vi "MODAQ RD v1.0 Main (DAQmx).vi"() -> ()   [LabVIEW 2019]
uses:
  Sub-VIs/Globals and Definitions/System Message.ctl
  <vilib>/Platform/TimedLoop/XDataNode/timing_clust.ctl
  <vilib>/Platform/TimedLoop/XDataNode/nitl_modes.ctl
  <vilib>/Platform/TimedLoop/XDataNode/wakeup.ctl
  Sub-VIs/Globals and Definitions/RT Globals RD v1.0.vi
  Sub-VIs/Globals and Definitions/Initialization Globals.vi
  Sub-VIs/Globals and Definitions/Control Globals RD v1.0.vi
  <instrlib>/niSync/niSync.llb/niSync Initialize (Default).vi
  <userlib>/_OpenG.lib/comparison/comparison.llb/U32 Changed__ogtk.vi
  <vilib>/Platform/TimedLoop/XDataNode/XDataNode.xnode
  <resource>/objmgr/nisysapi.rc
  <vilib>/Platform/TimedLoop/XDataNode/XDNodeRunTimeDep.lvlib
  <vilib>/nisyscfg/nisyscfg.lvlib
panel:
  in  "Port State":i32(ring)=3 items=["Disabled"=3, "Master"=6, "Passive"=7, "Slave"=9]
  out "Not SavingTDMS Data":bool
  out "Saving TDMS Data":bool=TRUE
  out "TDMS Recording Mode":string="Interval"
  out "Ring":u16(ring) items=["Fix Unavailable", "2D GNSS Fix", "3D GNSS Fix", "SBAS GNSS Fix", "Differential GNSS Fix", "Omnistar/Starfire GNSS fix", "RTK Float GNSS fix", "RTK Fixed GNSS fix"]
  out "GNSS Fix Status":i16
  out "PTP Time Server Found":bool
  out "satellites available":u8
  out "CPU Utili Label":string="CPU Utilization (%)"
  out "CPU Utilization %":string="3.4"
  out "RAM Free Label":string="RAM Free (%)"
  out "RAM Free (%)":string="88.0"
  out "Disk % Label":string="Disk Free (%)"
  out "Disk Free (%)":string="99.6"
  out "Disk Free Label":string="Disk Free (GB)"
  out "Disk Free (GB)":string="1992.8"
  out "Errors":errorcluster
  in  "STOP":bool
  out "Uptime String":string="Uptime:   0d  0h  0m"
  out "date/time string":string="Oct 26, 2023    12:39:58 UTC"
  out "Heading":string="Heading: 0.0°"
  out "Offset Distance":string="Offset: 11303146.1m"
  out "Current Position":string="Current Position: 0.000, 0.000"
  # "3 Phase Data Save"
  # "GPS Timekeeper Status"
  # "GPS Position Status"
  # "MODAQ\nNREL       RD v1.0"
  # "Public Reference\nDesign"
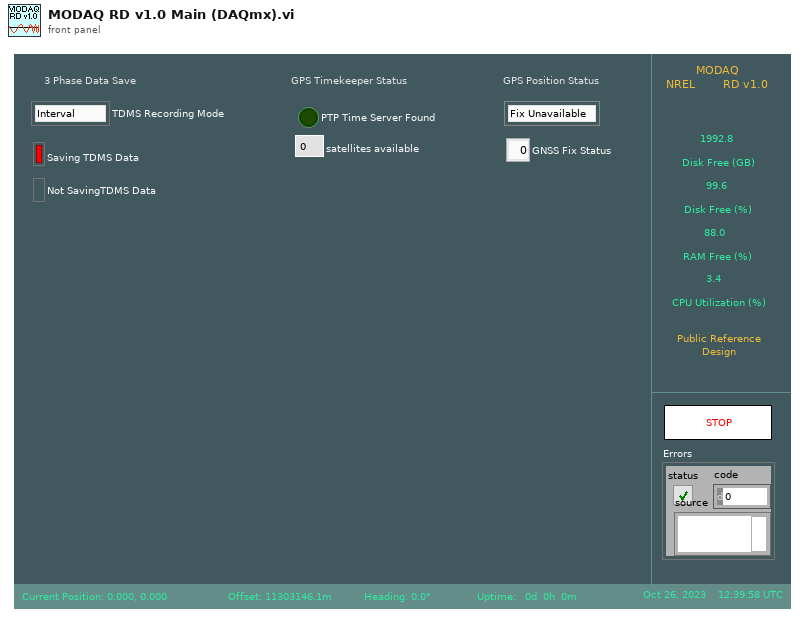
[diagram p1: front panel]
types:
  T1 = typedef "System Message.ctl" = cluster{"Message Tag":string, "Message Body":string, "Snooze Time (s)":dbl, "Snooze Alert?":bool, "Log Event?":bool, "Send Email":i32}
  T2 = typedef "All Tab Controls RDv1.0.ctl" = cluster{"Watch Circle":T3, "FTP and AWS":T4, "Email Settings":T5, "Summary File":T6, "File Settings":T7, "Watchdog":T9, "PowGrp0":T10, "Scaling Factors Grp0":dbl[], "PowGrp0 Sampling":cluster{"PowGrp0 sample rate [Hz]":dbl, "PowGrp0 samples per channel":i32}, "Stbd 3 Phase Voltage Scaling":dbl[], "Stbd 3 Phase Current Scaling":dbl[]}
  T3 = typedef "Watch Circle.ctl" = cluster{"Set Point Lat (dd)":dbl, "Set Point Lon (dd)":dbl, "Yellow Alert Radius (m)":dbl, "Red Alert Radius (m)":dbl, "AWOL Radius (m)":dbl, "Yellow Alert Snooze (min)":dbl, "Red Alert Snooze (min)":dbl, "AWOL Radius Snooze (min)":dbl}
  T4 = typedef "AWS and FTP.ctl" = cluster{"AWS Access Key":string, "AWS Secret Key":string, "AWS Bucket":string, "Enable AWS Upload (Summary)":bool, "Enable FTP Upload":bool, "FTP Host":string, "FTP User":string, "FTP Password":string, "Destination write path (pos)":string, "Local file path (pos)":string, "Summary  Upload Interval pos (min)":i32, "Delete Local File After Upload":bool, "Destination write path (pow)":string, "Local file path (pow)":string, "Summary Upload Interval pow (min)":i32, "Enable AWS Upload (TDMS)":bool}
  T5 = typedef "Email Settings.ctl" = cluster{"Enable Alerts":bool, "Distribution List (comma separated) 1":string, "Distribution List (comma separated) 2":string, "Sender Email":string, "SMTP":string, "Username":string, "Password":string}
  T6 = typedef "Summary File.ctl" = cluster{"Enable CSV":bool, "CSV Averaging Time (Sec)":i32, "CSV Loop Delay (ms)":i32}
  T7 = typedef "File Settings.ctl" = cluster{"Config File Path":string, "Data Folder Path":string, "Raw Mode":string, "Raw Interval (min)":i32, "Raw Sampling Time (min)":i32, "TDMS File Write Interval":T8, "Default Filename":path, "Enable TDMS Save (3ph only)":bool}
  T8 = typedef "Enum_FileNewInterval.ctl" = enum16{"10 Min", "Hourly", "Daily", "Weekly", "Monthly"}
  T9 = typedef "Watchdog.ctl" = cluster{"Watchdog Period (ms)":u32, "Reset System on WD timeout":bool, "Enable RT Watchdog":bool}
  T10 = typedef "TDMS Constants.ctl" = cluster{"Channel Names":string[], "Channel Units":string[], "TDMS File Suffix":string, "Channel Datatype":string[]}
  T11 = typedef "XDNodeRunTimeDep.lvlib/timing_clust.ctl" = cluster{"Expected End [f-1]":u64, "Actual End [f-1]":u64, "Finished Late? [f-1]":bool, "Expected End [i-1]":u64, "Actual End [i-1]":u64, "Finished Late? [i-1]":bool, "Expected Start [i]":u64, "Actual Start [i]":u64, "Expected Start [f]":u64, "Actual Start [f]":u64, "Source Name":string, "Structure Name":string, "Period":i64, "Deadline":i64, "Offset":i64, "Start":i64, "Priority":i32, "Timeout":i32, "Mode":T12, "Wakeup Reason":T13, "Error":errorcluster, "Source Type":string, "Secondary Source Type":string, "Global End Time":u64, "Global Start Time":u64, "Frame Duration":u64, "Iteration Duration":u64, "Assigned CPU":i32, "I/O Scan Engine Mode":u32}
  T12 = typedef "XDNodeRunTimeDep.lvlib/nitl_modes.ctl" = enum32{"No Change", "Process missed periods, maintain original phase", "Discard missed periods, maintain original phase", "Process missed periods, ignore original phase", "Discard missed periods, ignore original phase"}
  T13 = typedef "XDNodeRunTimeDep.lvlib/wakeup.ctl" = enum32{"Normal", "Aborted", "Asynchronous wakeup", "Timing source error", "Timed loop error", "Timeout"}
  T14 = enum16{"open", "replace", "create", "open or create", "replace or create", "replace or create with confirmation"}
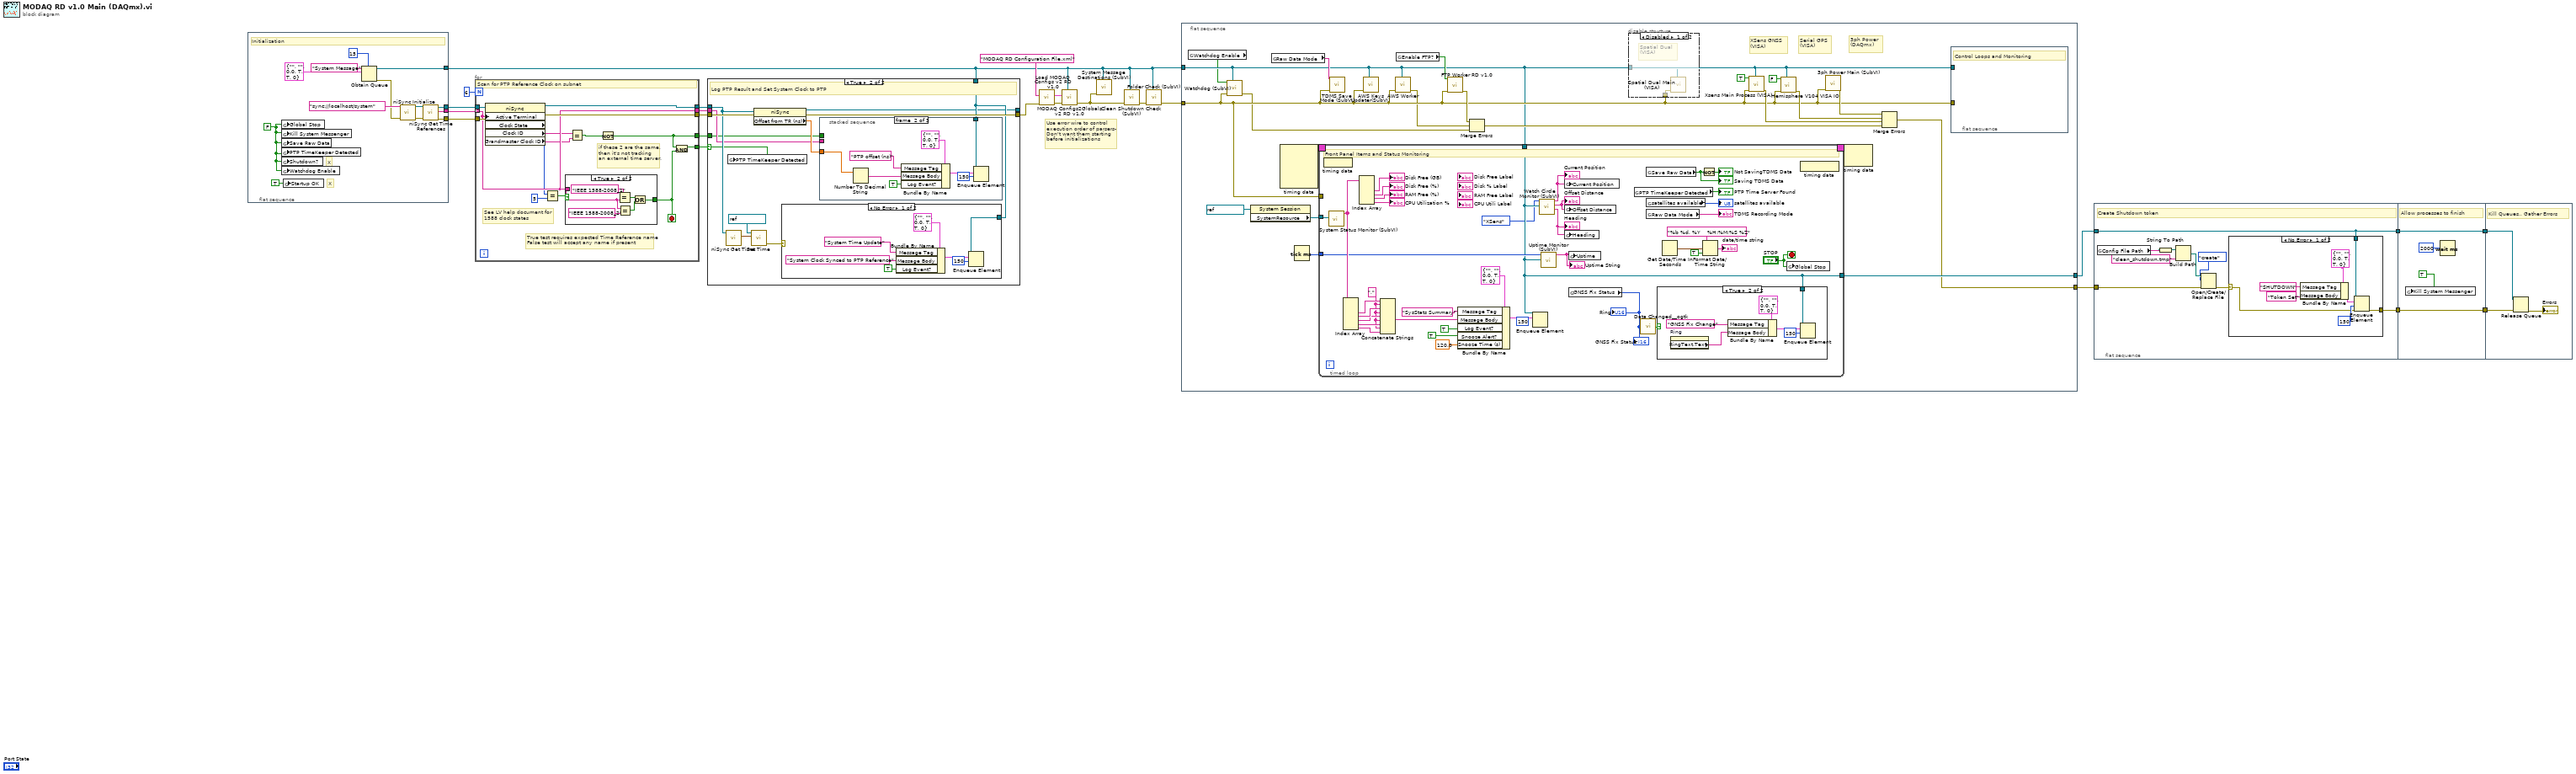
[diagram p0: block diagram]
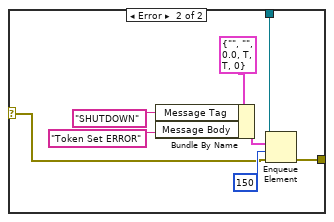
[diagram p4: hidden frame]
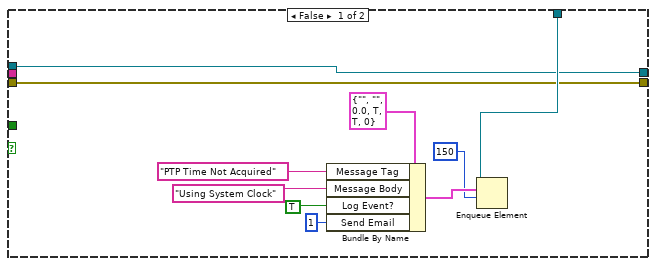
[diagram p5: hidden frame]
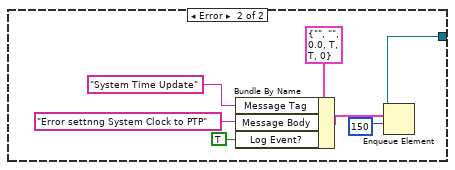
[diagram p6: hidden frame]
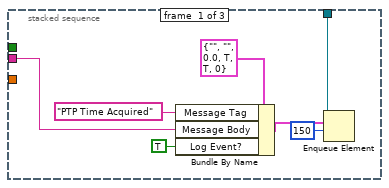
[diagram p7: hidden frame]
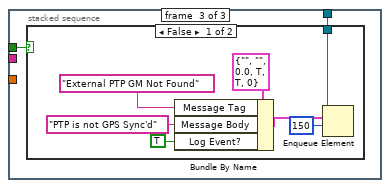
[diagram p8: hidden frame]
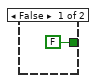
[diagram p10: hidden frame]
diagram:
  # "Use error wire to control\nexecution order of parsers-\nDon't want them starting\nbefore initializations"
  n1 = flat-sequence {
    tunnel: [w34] -> w11
    tunnel: [w26] -> w4
    tunnel: [w25] -> w5
    tunnel: [w24] -> w3
    frame #0 {
      w29 = FALSE ("Global_Stop")
      # "X"
      # "X"
      # "Initialization"
      n2 = global write "RT Globals RD v1.0.vi" "Global Stop"(w29) -> ()
      n3 = global write "RT Globals RD v1.0.vi" "Kill System Messenger"(w29) -> ()
      n4 = global write "Initialization Globals.vi" "Save Raw Data"(w29) -> ()
      n5 = global write "RT Globals RD v1.0.vi" "PTP TimeKeeper Detected"(w29) -> ()
      n6 = global write "Control Globals RD v1.0.vi" "Shutdown?"(w29) -> ()
      n7 = global write "Initialization Globals.vi" "Watchdog Enable"(w29) -> ()
      n8 = global write "Control Globals RD v1.0.vi" "Startup OK"(TRUE ("Startup OK")) -> ()
      n9 = Obtain Queue(max queue size (-1, unlimited)=15, name (unnamed)="System Message", element data type=T1 {"Message Tag"="", "Message Body"="", "Snooze Time (s)"=0.0, "Snooze Alert?"=TRUE, "Log Event?"=TRUE, "Send Email"=0}) -> (queue out=w34:refnum<queue>, error out=w30:errorcluster)  [unwired: 2 in, 1 out]
      n10 = call-poly <instrlib>:"niSync Initialize.vi"("error in (no error)"=w30, "resource name"=tag "sync://localhost/system") -> ("error out"=w27:errorcluster, "instrument handle out"=w28:refnum<k15>)  [unwired: 8 in]
      n11 = call <instrlib>:"niSync Get Time References.vi"("error in (no error)"=w27, "instrument handle"=w28) -> ("error out"=w26:errorcluster, "time references"=w24:string[], "instrument handle out"=w25:refnum<k15>)  [unwired: 7 in]
    }
  }
  n12 = for {
    N: 6 -> [_]
    tunnel: [w49] -> w19
    tunnel: [w47] -> w18
    tunnel: [w39] -> w17
    tunnel: w5 -> [w50]
    tunnel: w4 -> [w48]
    tunnel: w3 -> [w46] mode=indexing
    tunnel: [w46] -> w2
    tunnel: [w37] -> w1
    stop <- w38 stop-if-true
    # "See LV help document for 1588 clock states"
    # "if these 2 are the same, then it's not tracking\nan external time server."
    # "True test requires expected Time Reference name\nFalse test will accept any name if present"
    # "Scan for PTP Reference Clock on subnet"
    n13 = property class="niSync"(reference=w50, error in=w48, "Active Terminal"=w46) -> (reference out=w49:refnum<k15>, error out=w47:errorcluster, "Clock State"=w45:i32, "Clock ID"=w42:string, "Grandmaster Clock ID"=w41:string)
    n14 = Equal?(x=w45, y=5) -> (x = y?=w43:bool)
    n15 = case shown="True" w43 {
      tunnel: [FALSE w55] -> w38
      tunnel: w46 -> [_ w53]
      frame False {
      }
      frame True {
        n16 = Equal?(x="IEEE 1588-2008_1", y=w53) -> (x = y?=w57:bool)
        n17 = Equal?(x=w53, y="IEEE 1588-2008_2") -> (x = y?=w56:bool)
        n18 = Or(x=w57, y=w56) -> (x .or. y?=w55:bool)
      }
    }
    n19 = Equal?(x=w42, y=w41) -> (x = y?=w40:bool)
    n20 = Not(x=w40) -> (.not. x?=w37:bool)
    n21 = And(x=w37, y=w38) -> (x .and. y?=w39:bool)
  }
  n22 = case shown="True" w17 {
    selector: w17 -> [_ w69]
    tunnel: w11 -> [w62 w72]
    tunnel: w19 -> [w59 w75]
    tunnel: [w60 w79] -> w16
    tunnel: w18 -> [w60 w78]
    tunnel: [w59 w71] -> _
    tunnel: w2 -> [_ w70]
    tunnel: w1 -> [_ w68]
    frame False {
      n23 = Bundle By Name(cluster=T1 {"Message Tag"="", "Message Body"="", "Snooze Time (s)"=0.0, "Snooze Alert?"=TRUE, "Log Event?"=TRUE, "Send Email"=0}, "Message Tag"="PTP Time Not Acquired", "Message Body"="Using System Clock" ("Message Tag"), "Log Event?"=TRUE, "Send Email"=1) -> (w65:T1)
      n24 = Enqueue Element(queue=w62, element=w65, timeout in ms (-1)=150) -> ()  [unwired: 1 in, 3 out]
    }
    frame True {
      # "Log PTP Result and Set System Clock to PTP"
      n25 = call <instrlib>:"niSync Get Time.vi"("instrument handle"=w75) -> ("time"=w74:timestamp)  [unwired: 6 in, 2 out]
      n26 = global write "RT Globals RD v1.0.vi" "PTP TimeKeeper Detected"(w69) -> ()
      n27 = call <vilib>:"Set Time.vi"("Time"=w74, "Session in (localhost)"=refnum<k21> "localhost") -> ("error out"=w73:errorcluster)  [unwired: 6 in, 3 out]
      n28 = property class="niSync"(reference=w75, error in=w78) -> (reference out=w71:refnum<k15>, error out=w79:errorcluster, "Offset from TR (ns)"=w77:dbl)
      n29 = case shown="No Error" w73 {
        tunnel: w72 -> [w83 w88]
        frame No Error {
          n30 = Bundle By Name(cluster=T1 {"Message Tag"="", "Message Body"="", "Snooze Time (s)"=0.0, "Snooze Alert?"=TRUE, "Log Event?"=TRUE, "Send Email"=0}, "Message Tag"="System Time Update", "Message Body"="System Clock Synced to PTP Reference" ("Message Tag"), "Log Event?"=TRUE) -> (w85:T1)
          n31 = Enqueue Element(queue=w83, element=w85, timeout in ms (-1)=150) -> ()  [unwired: 1 in, 3 out]
        }
        frame Error {
          n32 = Bundle By Name(cluster=T1 {"Message Tag"="", "Message Body"="", "Snooze Time (s)"=0.0, "Snooze Alert?"=TRUE, "Log Event?"=TRUE, "Send Email"=0}, "Message Tag"="System Time Update", "Message Body"="Error settnng System Clock to PTP" ("Message Tag"), "Log Event?"=TRUE) -> (w92:T1)
          n33 = Enqueue Element(queue=w88, element=w92, timeout in ms (-1)=150) -> ()  [unwired: 1 in, 3 out]
        }
      }
      n34 = stacked-sequence {
        tunnel: w72 -> [w98 w106 w110]
        tunnel: w70 -> [w97 _ _]
        tunnel: w77 -> [_ w105 _]
        tunnel: w68 -> [_ _ w109]
        frame #0 {
          n35 = Bundle By Name(cluster=T1 {"Message Tag"="", "Message Body"="", "Snooze Time (s)"=0.0, "Snooze Alert?"=TRUE, "Log Event?"=TRUE, "Send Email"=0}, "Message Tag"="PTP Time Acquired", "Message Body"=w97, "Log Event?"=TRUE) -> (w99:T1)
          n36 = Enqueue Element(queue=w98, element=w99, timeout in ms (-1)=150) -> ()  [unwired: 1 in, 3 out]
        }
        frame #1 {
          n37 = Number To Decimal String(number=w105) -> (decimal integer string=w104:string)  [unwired: 1 in]
          n38 = Bundle By Name(cluster=T1 {"Message Tag"="", "Message Body"="", "Snooze Time (s)"=0.0, "Snooze Alert?"=TRUE, "Log Event?"=TRUE, "Send Email"=0}, "Message Tag"="PTP offset (ns)", "Message Body"=w104, "Log Event?"=TRUE) -> (w107:T1)
          n39 = Enqueue Element(queue=w106, element=w107, timeout in ms (-1)=150) -> ()  [unwired: 1 in, 3 out]
        }
        frame #2 {
          n40 = case shown="False" w109 {
            tunnel: w110 -> [w112 _]
            frame False {
              n41 = Bundle By Name(cluster=T1 {"Message Tag"="", "Message Body"="", "Snooze Time (s)"=0.0, "Snooze Alert?"=TRUE, "Log Event?"=TRUE, "Send Email"=0}, "Message Tag"="External PTP GM Not Found", "Message Body"="PTP is not GPS Sync'd", "Log Event?"=TRUE) -> (w116:T1)
              n42 = Enqueue Element(queue=w112, element=w116, timeout in ms (-1)=150) -> ()  [unwired: 1 in, 3 out]
            }
            frame True {
            }
          }
        }
      }
    }
  }
  n43 = call "Load MODAQ Configs v2 RD v1.0.vi"("error in (no error)"=w16, "MODAQ Config Filename"="MODAQ RD Configuration File.xml") -> ("error out"=w23:errorcluster, "Configs out"=w21:T2)  [unwired: 8 in]
  n44 = call "MODAQ Configs2Globals v2 RD v1.0.vi"("Configs in"=w21, "error in"=w23, "Queue in"=w11) -> ("error out"=w10:errorcluster)  [unwired: 7 in]
  n45 = call "System Message Destinations (SubVI).vi"("Queue in"=w11, "error in (no error)"=w10) -> ()  [unwired: 10 in]
  n46 = call "Clean Shutdown Check (SubVI).vi"("System Message Queue In"=w11, "error in (no error)"=w10) -> ("error out"=w12:errorcluster)  [unwired: 9 in]
  n47 = call "Folder Check (SubVI).vi"("System Message Queue In"=w11, "error in (no error)"=w12) -> ("error out"=w13:errorcluster)  [unwired: 9 in]
  n48 = flat-sequence {
    tunnel: w13 -> [w122]
    tunnel: w11 -> [w119]
    tunnel: [w126] -> w15
    tunnel: [w125] -> w14
    frame #0 {
      # "Serial GPS\n(VISA)"
      # "XSens GNSS\n(VISA)"
      # "3ph Power\n(DAQmx)"
      n49 = global read "Initialization Globals.vi" "Watchdog Enable"() -> (w118:bool)
      n50 = call "Watchdog (SubVI).vi"("System Message Queue In"=w119, "error in (no error)"=w122, "Enable Watchdog?"=w118) -> ("error out"=w121:errorcluster)  [unwired: 8 in]
      n51 = property class="System Session"(reference=refnum<k21> "localhost" ("System Session")) -> ("SystemResource"=w134:refnum<k20>)  [unwired: 1 in, 2 out]
      n52 = global read "Initialization Globals.vi" "Raw Data Mode"() -> (w135:string)
      n53 = node-c288() -> (w138:T11)  [unwired: 4 in]
      n54 = Tick Count (ms)() -> (millisecond timer value=w127:u32)
      n55 = timed-loop {
        timing: w138 -> [_]
        timing-out: [_] -> w137
        tunnel: w119 -> [w142]
        tunnel: w134 -> [w162]
        tunnel: w127 -> [w143]
        tunnel: [w142] -> w126
        tunnel: w122 -> [_]
        stop <- "STOP" stop-if-true
        w154 = ","
        (unwired) 150 ("timeout in ms (-1)")
        # "Front Panel Items and Status Monitoring"
        n56 = node-c288() -> ()  [unwired: 1 in]
        n57 = call "System Status Monitor (SubVI).vi"("Refnum in"=w162) -> ("System Status Array"=w146:string[])  [unwired: 8 in]
        n58 = Index Array(array=w146) -> (element #2=w159:string, element #3=w158:string, element #4=w157:string, element #5=w156:string, element #6=w155:string)  [unwired: 6 in, 1 out]
        n59 = Index Array(array=w146) -> (element #2=→"Disk Free (GB)":string, element #3=→"Disk Free (%)":string, element #4=→"RAM Free (%)":string, element #5=→"CPU Utilization %":string)  [unwired: 5 in, 1 out]
        n60 = Concatenate Strings(w159, w154, w158, w154, w157, w154, w156, w154, w155) -> (w153:string)
        n61 = Bundle By Name(cluster=T1 {"Message Tag"="", "Message Body"="", "Snooze Time (s)"=0.0, "Snooze Alert?"=TRUE, "Log Event?"=TRUE, "Send Email"=0}, "Message Tag"="SysStats Summary", "Message Body"=w153, "Log Event?"=TRUE, "Snooze Alert?"=TRUE, "Snooze Time (s)"=120.0) -> (w161:T1)
        n62 = Enqueue Element(queue=w142, element=w161) -> ()  [unwired: 2 in, 3 out]
        n63 = call "Watch Circle Monitor (SubVI).vi"("Queue in"=w142, "GPS Source"=enum16{"Spatial Dual", "V104", "XSens"}."XSens") -> ("Heading"=w148:string, "Offset Distance"=w149:string, "Current Position"=w150:string)  [unwired: 7 in]
        "Current Position" <- w150
        "Offset Distance" <- w149
        "Heading" <- w148
        n64 = call "Uptime Monitor (SubVI).vi"("Queue in"=w142, "Start ms"=w143) -> ("Uptime String"=w147:string)  [unwired: 9 in]
        "Uptime String" <- w147
        n65 = global write "RT Globals RD v1.0.vi" "Current Position"(w150) -> ()
        n66 = global write "RT Globals RD v1.0.vi" "Offset Distance"(w149) -> ()
        n67 = global write "RT Globals RD v1.0.vi" "Heading"(w148) -> ()
        n68 = global write "RT Globals RD v1.0.vi" "Uptime"(w147) -> ()
        n69 = global read "RT Globals RD v1.0.vi" "GNSS Fix Status"() -> (w173:u32)
        "Ring" <- w173
        "GNSS Fix Status" <- w173
        n70 = global read "RT Globals RD v1.0.vi" "PTP TimeKeeper Detected"() -> (→"PTP Time Server Found":bool)
        n71 = call-poly <userlib>:"Data Changed__ogtk.vi"("U32"=w173) -> ("Changed"=w172:bool)
        n72 = global read "Initialization Globals.vi" "Save Raw Data"() -> (w177:bool)
        "Saving TDMS Data" <- w177
        n73 = global read "RT Globals RD v1.0.vi" "satellites available"() -> (→"satellites available":u8)
        n74 = global read "Initialization Globals.vi" "Raw Data Mode"() -> (→"TDMS Recording Mode":string)
        n75 = case shown="True" w172 {
          tunnel: w142 -> [_ w183]
          frame False {
          }
          frame True {
            n76 = property on="Ring" class="Ring (strict)"() -> ("RingText.Text"=w182:string)  [unwired: 2 in, 2 out]
            n77 = Bundle By Name(cluster=T1 {"Message Tag"="", "Message Body"="", "Snooze Time (s)"=0.0, "Snooze Alert?"=TRUE, "Log Event?"=TRUE, "Send Email"=0}, "Message Tag"="GNSS Fix Change", "Message Body"=w182) -> (w184:T1)
            n78 = Enqueue Element(queue=w183, element=w184, timeout in ms (-1)=150) -> ()  [unwired: 1 in, 3 out]
          }
        }
        n79 = Get Date/Time In Seconds() -> (seconds since 1Jan1904=w168:timestamp)
        n80 = Not(x=w177) -> (.not. x?=→"Not SavingTDMS Data":bool)
        n81 = Format Date/Time String(time format string (%c)="%b %d, %Y    %H:%M:%S %Z", seconds (now)=w168, UTC format=TRUE) -> (date/time string=→"date/time string":string)
        n82 = global write "RT Globals RD v1.0.vi" "Global Stop"("STOP") -> ()
        n83 = node-c288() -> ()  [unwired: 1 out]
      }
      n84 = call "TDMS Save Mode (SubVI).vi"("error in (no error)"=w122, "Raw Data Mode"=w135) -> ()  [unwired: 10 in]
      n85 = call "AWS Keys Updater(SubVI).vi"("Queue in"=w119, "error in (no error)"=w122) -> ()  [unwired: 10 in]
      n86 = call "AWS Worker.vi"("System Message Queue In"=w119, "error in (no error)"=w122) -> ("error out"=w120:errorcluster)  [unwired: 9 in]
      n87 = global read "Initialization Globals.vi" "Enable FTP?"() -> (w131:bool)
      n88 = call "FTP Worker RD v1.0.vi"("error in (no error)"=w122, "Enable FTP?"=w131) -> ("error out"=w133:errorcluster)  [unwired: 9 in]
      n89 = Merge Errors(w133, w120, w121) -> (w128:errorcluster)
      n90 = disable-structure shown="Disabled" {
        disable-tunnel: w119 -> [w140 _]
        disable-tunnel: w122 -> [w139 _]
        frame Disabled {
          # "Spatial Dual\n(VISA)"
          n91 = call "Spatial Dual Main (VISA).vi"("Queue in"=w140, "error in"=w139) -> ()  [unwired: 8 in, 1 out]
        }
        frame Enabled {
        }
      }
      n92 = call "Xsens Main Process (VISA).vi"("Sys Msg Queue"=w119, "error in (no error)"=w122, "Xsens Enable?"=TRUE) -> ("error out"=w129:errorcluster)  [unwired: 8 in]
      n93 = call "Hemisphere V104 VISA IO.vi"("Sys Msg Queue"=w119, "error in (no error)"=w122, "Enabled?"=FALSE) -> ("error out"=w130:errorcluster)  [unwired: 8 in]
      n94 = call "3ph Power Main (SubVI).vi"("error in (no error)"=w122) -> ("error out"=w132:errorcluster)  [unwired: 10 in]
      n95 = node-c288(w137) -> ()  [unwired: 1 out]
      n96 = Merge Errors(w132, w130, w129, w128) -> (w125:errorcluster)
      n97 = flat-sequence {
        tunnel: w122 -> [_]
        tunnel: w119 -> [_]
        frame #0 {
          # "Control Loops and Monitoring"
        }
      }
    }
  }
  n98 = flat-sequence {
    tunnel: [w190] -> w9
    tunnel: [w189] -> w7
    tunnel: w15 -> [w190]
    tunnel: w14 -> [w192]
    tunnel: w9 -> [w217]
    tunnel: [w217] -> w8
    tunnel: w7 -> [w216]
    tunnel: [w216] -> w6
    tunnel: w8 -> [w218]
    tunnel: w6 -> [w219]
    frame #0 {
      # "Create Shutdown token"
      n99 = global read "Initialization Globals.vi" "Config File Path"() -> (w196:string)
      n100 = String To Path(string=w196) -> (path=w195:path)
      n101 = Build Path(base path=w195, name or relative path="clean_shutdown.tmp") -> (appended path=w197:path)
      n102 = Open/Create/Replace File(file path (use dialog)=w197, error in=w192, operation (0:open)=T14."create") -> (error out=w191:errorcluster)  [unwired: 3 in, 2 out]
      n103 = case shown="No Error" w191 {
        selector: w191 -> [w203 w206]
        tunnel: w190 -> [w205 w208]
        tunnel: [w200 w207] -> w189
        frame No Error {
          n104 = Bundle By Name(cluster=T1 {"Message Tag"="", "Message Body"="", "Snooze Time (s)"=0.0, "Snooze Alert?"=TRUE, "Log Event?"=TRUE, "Send Email"=0}, "Message Tag"="SHUTDOWN", "Message Body"="Token Set") -> (w202:T1)
          n105 = Enqueue Element(queue=w205, element=w202, timeout in ms (-1)=150, error in (no error)=w203) -> (error out=w200:errorcluster)  [unwired: 2 out]
        }
        frame Error {
          n106 = Bundle By Name(cluster=T1 {"Message Tag"="", "Message Body"="", "Snooze Time (s)"=0.0, "Snooze Alert?"=TRUE, "Log Event?"=TRUE, "Send Email"=0}, "Message Tag"="SHUTDOWN", "Message Body"="Token Set ERROR") -> (w212:T1)
          n107 = Enqueue Element(queue=w208, element=w212, timeout in ms (-1)=150, error in (no error)=w206) -> (error out=w207:errorcluster)  [unwired: 2 out]
        }
      }
    }
    frame #1 {
      # "Allow processes to finish"
      n108 = global write "RT Globals RD v1.0.vi" "Kill System Messenger"(TRUE ("Kill System Messenger")) -> ()
      n109 = Wait (ms)(milliseconds to wait=u32 2000) -> ()  [unwired: 1 out]
    }
    frame #2 {
      # "Kill Queues,, Gather Errors"
      n110 = Release Queue(queue=w218, error in (no error)=w219) -> (error out=→"Errors":errorcluster)  [unwired: 1 in, 2 out]
    }
  }
